vi "采集结束.vi"() -> ()   [LabVIEW 2013]
panel:
  in  "采集结束":bool
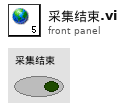
[diagram p1: front panel]
diagram:
